vi "Main.vi"(11 "Module Admin":refnum<class "Delacor_lib_QMH_Module Admin.lvclass">) -> ()   [LabVIEW 2020, in "Acquisition.lvlib"]
doc: "This template is based off of the Queued Message Handler design pattern and the Queued Message Handler project template that ships with LabVIEW.\n\nThe main difference is that the queue is private to this module and communication between modules is performed via Broadcast and Request events.\n\nRequest events are wrapped in public API methods and are handled in the Event Handling Loop (EHL) of this VI. Any module can register for Broadcast events sent by this module. The EHL generates messages based on user interface actions.\n\nThe Message Handling Loop (MHL) processes messages generated by the EHL, or by other messages. The messages are string values, so new messages can be added easily to the Message Cases case structure in the MHL. Each message cluster can also provide an optional value for Message Data, which is a variant that can be converted to whatever message-specific data is required.\n_____\nBased on Delacor QMH Project Template 5.0.0.82."
uses:
  Acquisition.lvlib
  <vilib>/Delacor/Delacor QMH/Libraries/Module Admin_class/Delacor_lib_QMH_Module Admin.lvclass
  Module Data--cluster.ctl
  Stop Helper Loop Argument--cluster.ctl
  Stop Argument--cluster.ctl
  <vilib>/Delacor/Delacor QMH/Libraries/Message Queue_class/Delacor_lib_QMH_Message Queue.lvclass/Delacor_lib_QMH_Message Queue.ctl
  <vilib>/Delacor/Delacor QMH/Libraries/Module Admin_class/Delacor_lib_QMH_Module Admin.lvclass/Delacor_lib_QMH_Module Admin.ctl
  Start Acquire Argument--cluster.ctl
  Stop Acquire Argument--cluster.ctl
  <vilib>/Utility/miscctls.llb/LVPointTypeDef.ctl
  <vilib>/Delacor/Delacor QMH/Libraries/Message Queue_class/Delacor_lib_QMH_Enqueue Message (Single).vi
  <vilib>/Delacor/Delacor QMH/Libraries/Module Admin_class/Delacor_lib_QMH_Get External Launch.vi
  <vilib>/Utility/error.llb/Error Cluster From Error Code.vi
  <vilib>/ErrorRing/Error Ring.xnode
  <vilib>/Delacor/Delacor QMH/Libraries/Message Queue_class/Delacor_lib_QMH_Message Queue.lvclass
panel:
  out "Waveform Graph":dynamicdata(graph)
  out "error out":errorcluster
  out "Status":string
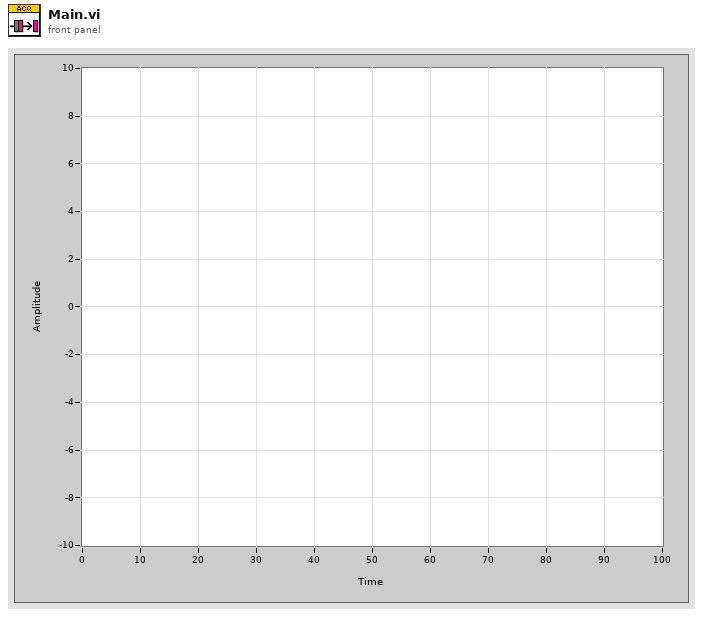
[diagram p1: front panel]
types:
  T1 = typedef "Acquisition.lvlib/Request Events--cluster.ctl" = cluster{"Stop Module":refnum<user-event>, "Show Panel":refnum<user-event>, "Hide Panel":refnum<user-event>, "Get Module Execution Status":refnum<user-event>, "Show Diagram":refnum<user-event>, "Start Helper Loop":refnum<user-event>, "Stop Helper Loop":refnum<user-event>, "Start Acquire":refnum<user-event>, "Stop Acquire":refnum<user-event>}
  T2 = typedef "Acquisition.lvlib/Module Data--cluster.ctl" = cluster{"Status":string}
  T3 = typedef "Acquisition.lvlib/Stop Helper Loop Argument--cluster.ctl" = cluster{"Boolean":bool}
  T4 = enum32{"invalid lock state", "Not Locked", "Locked (No Password)", "Password-protected"}
  T5 = typedef "Acquisition.lvlib/Stop Argument--cluster.ctl" = cluster{"Origin":string, "Exit via Stop Module Req?":bool, "Wait for Module to stop?":bool}
  T6 = typedef "Acquisition.lvlib/Start Acquire Argument--cluster.ctl" = cluster{"Boolean":bool}
  T7 = typedef "Acquisition.lvlib/Stop Acquire Argument--cluster.ctl" = cluster{"Boolean":bool}
  T8 = typedef "LVPointTypeDef.ctl" = cluster{"Horizontal":i16, "Vertical":i16}
  T9 = enum32{"Invalid", "Standard", "Closed", "Hidden", "Minimized", "Maximized"}
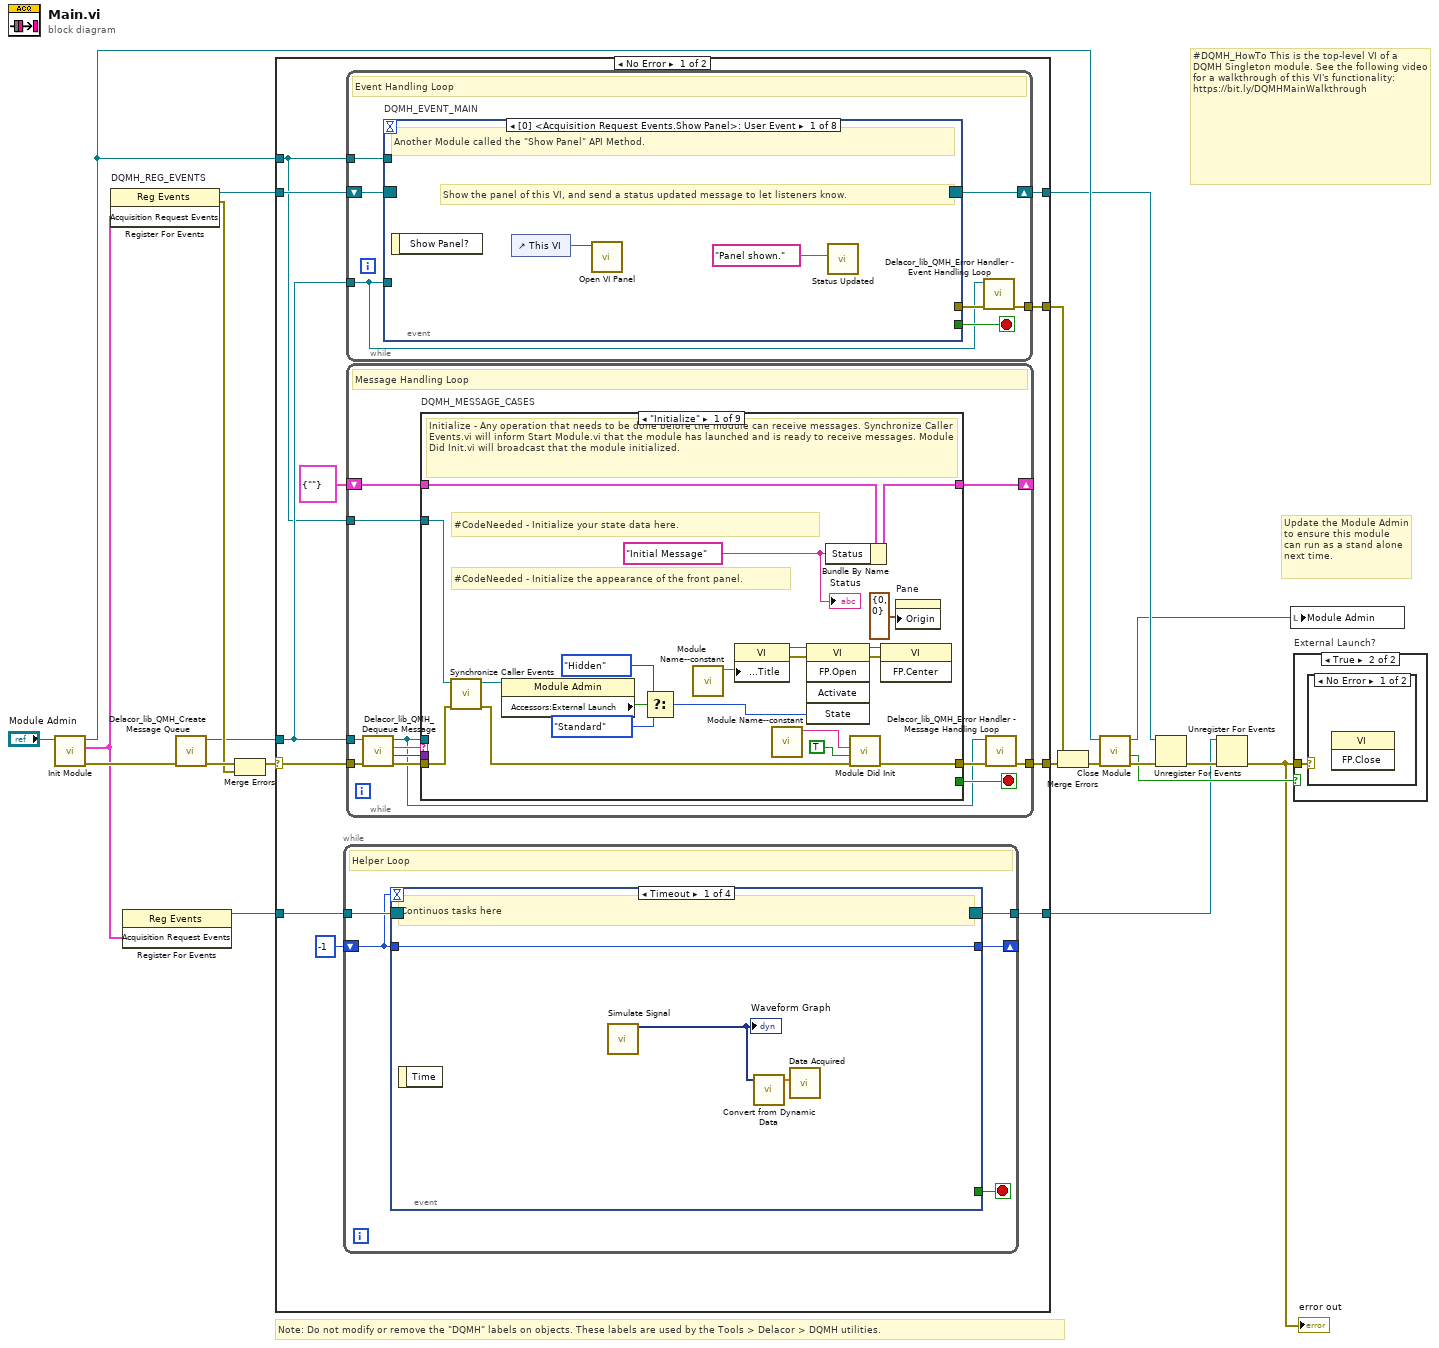
[diagram p0: block diagram]
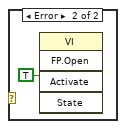
[diagram p3: hidden frame]
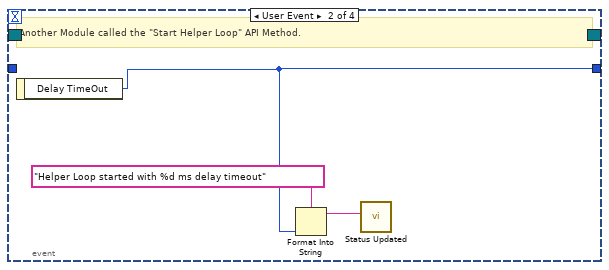
[diagram p4: hidden frame]
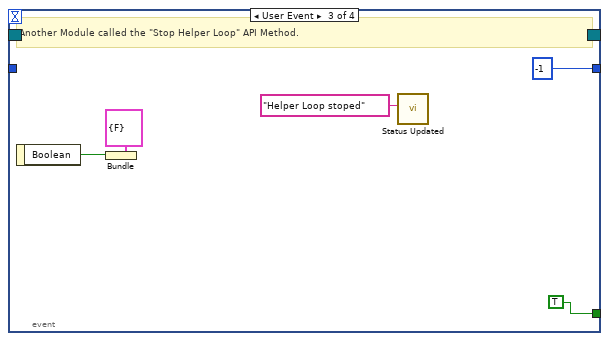
[diagram p5: hidden frame]
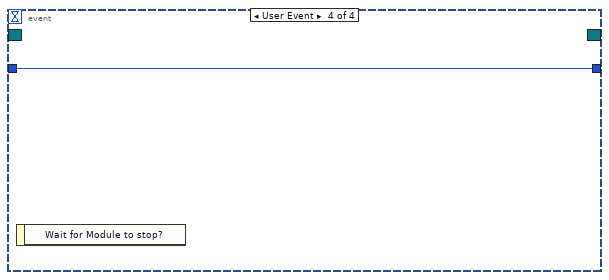
[diagram p6: hidden frame]
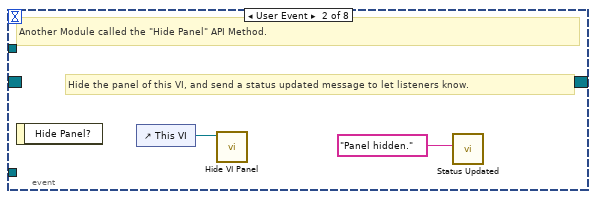
[diagram p7: hidden frame]
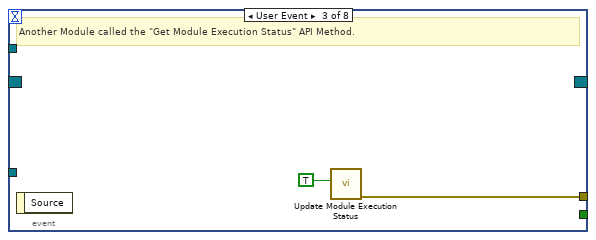
[diagram p8: hidden frame]
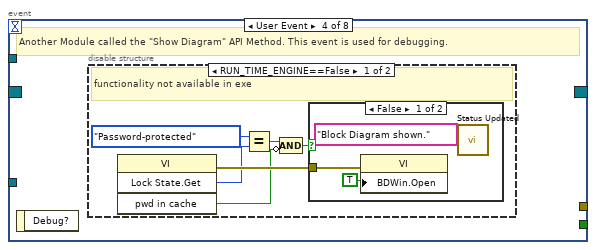
[diagram p9: hidden frame]
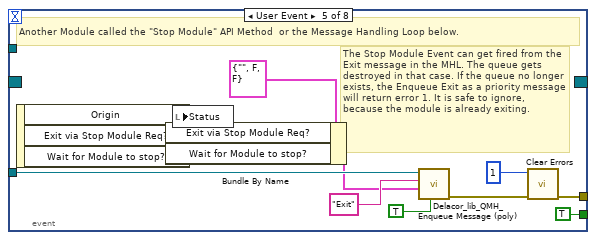
[diagram p12: hidden frame]
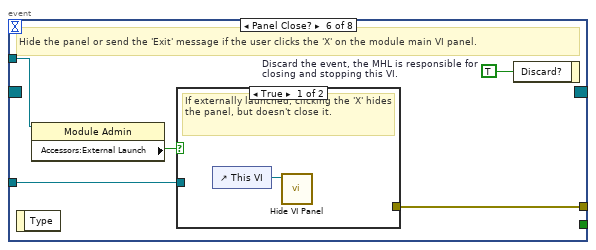
[diagram p13: hidden frame]
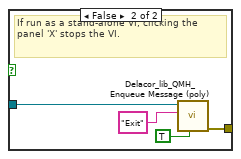
[diagram p14: hidden frame]
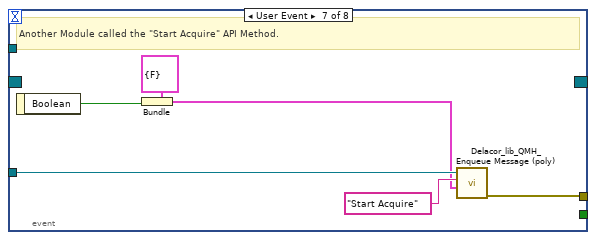
[diagram p15: hidden frame]
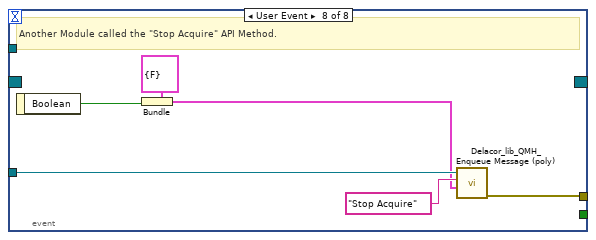
[diagram p16: hidden frame]
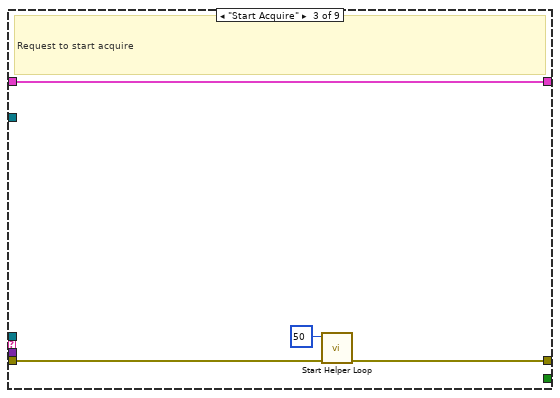
[diagram p18: hidden frame]
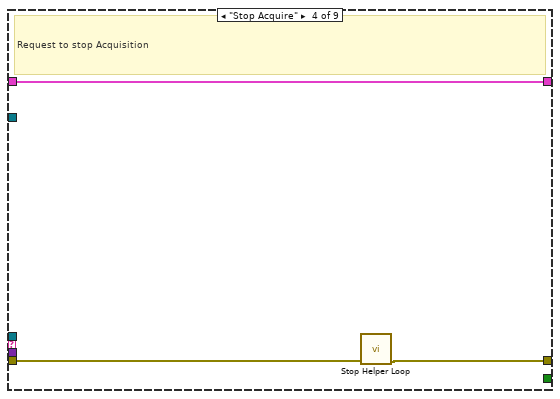
[diagram p19: hidden frame]
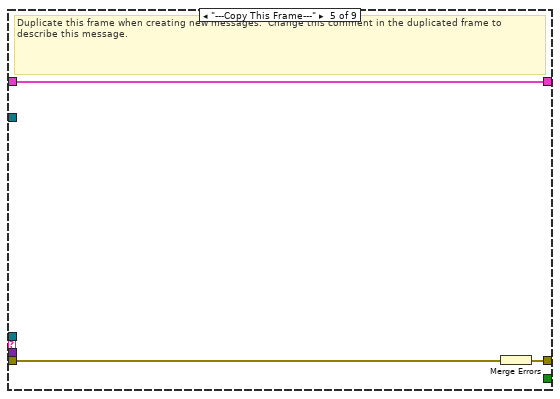
[diagram p20: hidden frame]
diagram:
  # "#DQMH_HowTo This is the top-level VI of a DQMH Singleton module. See the following video for a walkthrough of this VI's functionality: https://bit.ly/DQMHMainWalkthrough"
  # "Note: Do not modify or remove the \"DQMH\" labels on objects. These labels are used by the Tools > Delacor > DQMH utilities."
  # "Update the Module Admin to ensure this module can run as a stand alone next time."
  n1 = call "Init Module.vi"("Singleton Module Admin in"="Module Admin") -> ("error out"=w19:errorcluster, "Acquisition Request Events"=w3:T1, "Singleton Module Admin out"=w11:refnum<class "Delacor_lib_QMH_Module Admin.lvclass">)  [unwired: 8 in]
  n2 = register-events "DQMH_REG_EVENTS"(w3) -> (reference out=w9:refnum<event-registration>, error out=w12:errorcluster)  [unwired: 2 in]
  n3 = register-events(w3) -> (reference out=w4:refnum<event-registration>)  [unwired: 2 in, 1 out]
  n4 = call <vilib>:"Delacor_lib_QMH_Create Message Queue.vi"("error in (no error)"=w19) -> ("error out"=w14:errorcluster, "Message Queue"=w8:refnum<class "Delacor_lib_QMH_Message Queue.lvclass">)  [unwired: 9 in]
  n5 = Merge Errors(w14, w12) -> (w13:errorcluster)
  n6 = case shown="No Error" w13 {
    selector: w13 -> [w29 w199]
    tunnel: [w31 w198] -> w20
    tunnel: [w28 w204] -> w10
    tunnel: w9 -> [w26 w204]
    tunnel: w8 -> [w25 w197]
    tunnel: [w30 _] -> w17
    tunnel: w11 -> [w24 w200]
    tunnel: w4 -> [w23 _]
    tunnel: [w22 _] -> w1
    frame No Error {
      n7 = while {
        tunnel: w23 -> [w36]
        tunnel: [w35] -> w22
        shift-right: [w34] -> _
        shift-left: -1 -> [w33]
        stop <- w32 stop-if-true
        # "Helper Loop"
        n8 = event shown="[0] Timeout" {
          selector: w36 -> [_ _ _ _]
          dyn-events: [_ _ _ _] -> w35
          timeout: w33 -> [_ _ _ _]
          tunnel: [w39 w41 -1 w48] -> w34
          tunnel: w33 -> [w39 _ _ w48]
          tunnel: [_ _ TRUE _] -> w32
          event Timeout {
            # "Continuos tasks here"
            n9 = event-data() -> ()  [unwired: 1 in, 1 out]
            n10 = call "Simulate Signal"() -> ("Sine"=w38:dynamicdata)  [unwired: 14 in, 1 out]
            "Waveform Graph" <- w38
            n11 = call "Convert from Dynamic Data"("Dynamic Data Type"=w38) -> ("Array"=w37:dbl[])  [unwired: 3 in]
            n12 = call "Data Acquired.vi"("Data"=w37) -> ()  [unwired: 10 in, 1 out]
          }
          event User Event {
            # "Another Module called the \"Start Helper Loop\" API Method."
            n13 = event-data() -> ("Delay TimeOut"=w41:i32)  [unwired: 1 in]
            n14 = Format Into String(format string="Helper Loop started with %d ms delay timeout", w41) -> (resulting string=w42:string)  [unwired: 2 in, 1 out]
            n15 = call "Status Updated.vi"("Status"=w42) -> ()  [unwired: 10 in, 1 out]
          }
          event User Event {
            # "Another Module called the \"Stop Helper Loop\" API Method."
            n16 = event-data() -> ("Boolean"=w46:bool)  [unwired: 1 in]
            n17 = Bundle(cluster=T3 {"Boolean"=FALSE} ("Stop Helper Loop Argument"), "Boolean"=w46) -> ()  [unwired: 1 out]
            n18 = call "Status Updated.vi"("Status"="Helper Loop stoped") -> ()  [unwired: 10 in, 1 out]
          }
          event User Event {
            n19 = event-data() -> ()  [unwired: 1 in, 1 out]
          }
        }
      }
      n20 = while {
        tunnel: w25 -> [w49]
        shift-right: [w52] -> w28
        shift-left: w26 -> [w53]
        tunnel: [w54] -> w30
        tunnel: w24 -> [w50]
        stop <- w51 stop-if-true
        # "Event Handling Loop"
        n21 = event "DQMH_EVENT_MAIN" shown="[0] <Acquisition Request Events.Show Panel>: User Event" {
          selector: w53 -> [_ _ _ _ _ _ _ _]
          dyn-events: [_ _ _ _ _ _ _ _] -> w52
          timeout: _ -> [_ _ _ _ _ _ _ _]
          tunnel: [_ _ _ _ TRUE ("Discard?") _ _ _] -> w51
          tunnel: w49 -> [_ _ _ _ w78 w85 w98 w104]
          tunnel: [_ _ w61 _ w81 w87 w93 w99] -> w55
          tunnel: w50 -> [_ _ _ _ _ w84 _ _]
          event User Event {
            # "Show the panel of this VI, and send a status updated message to let listeners know."
            # "Another Module called the \"Show Panel\" API Method."
            n22 = event-data() -> ()  [unwired: 1 in, 1 out]
            n23 = control-ref of="This VI"() -> (w57:refnum<vi>)
            n24 = call "Open VI Panel.vi"("VI"=w57) -> ()  [unwired: 10 in, 1 out]
            n25 = call "Status Updated.vi"("Status"="Panel shown." ("format string")) -> ()  [unwired: 10 in, 1 out]
          }
          event User Event {
            # "Hide the panel of this VI, and send a status updated message to let listeners know."
            # "Another Module called the \"Hide Panel\" API Method."
            n26 = event-data() -> ()  [unwired: 1 in, 1 out]
            n27 = control-ref of="This VI"() -> (w59:refnum<vi>)
            n28 = call "Hide VI Panel.vi"("VI"=w59) -> ()  [unwired: 10 in, 1 out]
            n29 = call "Status Updated.vi"("Status"="Panel hidden." ("format string")) -> ()  [unwired: 10 in, 1 out]
          }
          event User Event {
            # "Another Module called the \"Get Module Execution Status\" API Method."
            n30 = event-data() -> ()  [unwired: 1 in, 1 out]
            n31 = call "Update Module Execution Status.vi"("Running?"=TRUE) -> ("error out"=w61:errorcluster)  [unwired: 10 in]
          }
          event User Event {
            # "Another Module called the \"Show Diagram\" API Method. This event is used for debugging."
            n32 = event-data() -> ()  [unwired: 1 in, 1 out]
            n33 = disable-structure shown="RUN_TIME_ENGINE==False" {
              frame condition #0 (active) {
                # "functionality not available in exe"
                n34 = invoke class="VI" method="Lock State.Get"() -> (error out=w67:errorcluster, "Get Lock State"=w66:T4, "pwd in cache"=w63:bool)  [unwired: 4 in, 1 out]
                n35 = Equal?(x=T4."Password-protected", y=w66) -> (x = y?=w64:bool)
                n36 = Compound Arithmetic op=AND(w64, invert w63) -> (w62:bool)
                n37 = case shown="False" w62 {
                  tunnel: w67 -> [w70 _]
                  frame False {
                    n38 = property class="VI"(error in=w70, "BDWin.Open"=TRUE ("Block Diagram Window:Open")) -> ()  [unwired: 1 in, 2 out]
                    n39 = call "Status Updated.vi"("Status"="Block Diagram shown." ("format string")) -> ()  [unwired: 10 in, 1 out]
                  }
                  frame True {
                    # "Password-protected VI, and the password is not in the cache. Do not show the diagram."
                  }
                }
              }
              frame condition #1 {
              }
            }
          }
          event User Event {
            # "The Stop Module Event can get fired from the Exit message in the MHL. The queue gets destroyed in that case. If the queue no longer exists, the Enqueue Exit as a priority message will return error 1. It is safe to ignore, because the module is already exiting."
            # "Another Module called the \"Stop Module\" API Method  or the Message Handling Loop below."
            n40 = event-data() -> ("Origin"=w77:string, "Exit via Stop Module Req?"=w73:bool, "Wait for Module to stop?"=w72:bool)  [unwired: 1 in]
            n41 = Bundle By Name(cluster=T5 {"Origin"="", "Exit via Stop Module Req?"=FALSE, "Wait for Module to stop?"=FALSE} ("Stop Argument"), "Exit via Stop Module Req?"=w73, "Wait for Module to stop?"=w72) -> (w71:T5)
            n42 = local write "Status"(w77) -> ()
            n43 = call-poly <vilib>:"Delacor_lib_QMH_Enqueue Message (poly).vi"("Priority Message? (F)"=TRUE, "Message Data"=w71, "Message"="Exit", "Message Queue in"=w78) -> ("error out"=w82:errorcluster)  [unwired: 6 in, 1 out]
            n44 = call <vilib>:"Clear Errors.vi"("error in (no error)"=w82, "specific error code to clear (0: all)"=1) -> ("error out"=w81:errorcluster)  [unwired: 4 in, 1 out]
          }
          event Panel Close? {
            w86 = TRUE  # Discard the event, the MHL is responsible for closing and stopping this VI.
            # "Hide the panel or send the 'Exit' message if the user clicks the 'X' on the module main VI panel."
            n45 = event-data() -> ()  [unwired: 1 in, 1 out]
            n46 = property class="Module Admin"(reference=w84) -> ("Accessors:External Launch"=w83:bool)  [unwired: 1 in, 2 out]
            n47 = case shown="True" w83 {
              tunnel: w85 -> [_ w91]
              tunnel: [_ w92] -> w87
              frame True {
                # "If externally launched, clicking the 'X' hides the panel, but doesn't close it."
                n48 = control-ref of="This VI"() -> (w88:refnum<vi>)
                n49 = call "Hide VI Panel.vi"("VI"=w88) -> ()  [unwired: 10 in, 1 out]
              }
              frame False {
                # "If run as a stand-alone VI, clicking the panel 'X' stops the VI."
                n50 = call-poly <vilib>:"Delacor_lib_QMH_Enqueue Message (poly).vi"("Priority Message? (F)"=TRUE, "Message"="Exit", "Message Queue in"=w91) -> ("error out"=w92:errorcluster)  [unwired: 7 in, 1 out]
              }
            }
            n51 = event-data("Discard?"=w86) -> ()  [unwired: 1 in, 1 out]
          }
          event User Event {
            # "Another Module called the \"Start Acquire\" API Method."
            n52 = event-data() -> ("Boolean"=w94:bool)  [unwired: 1 in]
            n53 = Bundle(cluster=T6 {"Boolean"=FALSE} ("Start Acquire Argument"), "Boolean"=w94) -> (w95:T6)
            n54 = call-poly <vilib>:"Delacor_lib_QMH_Enqueue Message (poly).vi"("Message Data"=w95, "Message"="Start Acquire", "Message Queue in"=w98) -> ("error out"=w93:errorcluster)  [unwired: 7 in, 1 out]
          }
          event User Event {
            # "Another Module called the \"Stop Acquire\" API Method."
            n55 = event-data() -> ("Boolean"=w100:bool)  [unwired: 1 in]
            n56 = Bundle(cluster=T7 {"Boolean"=FALSE} ("Stop Acquire Argument"), "Boolean"=w100) -> (w101:T7)
            n57 = call-poly <vilib>:"Delacor_lib_QMH_Enqueue Message (poly).vi"("Message Data"=w101, "Message"="Stop Acquire", "Message Queue in"=w104) -> ("error out"=w99:errorcluster)  [unwired: 7 in, 1 out]
          }
        }
        n58 = call-dynamic "Delacor_lib_QMH_Error Handler - Event Handling Loop.vi"("error in (no error)"=w55, "Message Queue in"=w49) -> ("dup error in"=w54:errorcluster)  [unwired: 8 in, 1 out]
      }
      n59 = while {
        tunnel: w25 -> [w107]
        shift-right: [w111] -> _
        shift-left: T2 {"Status"=""} ("Data Cluster") -> [w112]
        tunnel: w29 -> [w115]
        tunnel: [w113] -> w31
        tunnel: w24 -> [w105]
        stop <- w110 stop-if-true
        # "Message Handling Loop"
        n60 = call-dynamic "Delacor_lib_QMH_Dequeue Message.vi"("error in (no error)"=w115, "Message Queue in"=w107) -> ("error out"=w114:errorcluster, "Message Data"=w108:variant, "Message"=w109:string, "Message Queue out"=w106:refnum<class "Delacor_lib_QMH_Message Queue.lvclass">)  [unwired: 6 in]
        n61 = case "DQMH_MESSAGE_CASES" shown="\"Initialize\"" w109 {
          selector: w109 -> [_ _ _ _ _ _ _ _ w184]
          tunnel: w106 -> [_ _ _ _ _ _ w154 w176 _]
          tunnel: w114 -> [w134 w138 w141 w144 w148 w150 w161 w182 w186]
          tunnel: [w132 w138 w140 w143 w147 w150 w157 w179 w187] -> w116
          tunnel: w112 -> [w123 w137 w142 w145 w146 w149 w156 w175 w185]
          tunnel: [w122 w137 w142 w145 w146 w149 w156 w175 w185] -> w111
          tunnel: [_ _ _ _ _ _ _ w174 _] -> w110
          tunnel: w108 -> [_ _ _ _ _ _ w155 w173 _]
          tunnel: w105 -> [w124 _ _ _ _ _ w153 w168 _]
          frame "Initialize" {
            w117 = "Initial Message" ("Initial Message")
            # "#CodeNeeded - Initialize the appearance of the front panel."
            # "#CodeNeeded - Initialize your state data here."
            # "Initialize - Any operation that needs to be done before the module can receive messages. Synchronize Caller Events.vi will inform Start Module.vi that the module has launched and is ready to receive messages. Module Did Init.vi will broadcast that the module initialized."
            n62 = call "Synchronize Caller Events.vi"("error in (no error)"=w134, "Singleton Module Admin in"=w124) -> ("error out"=w133:errorcluster, "Singleton Module Admin out"=w119:refnum<class "Delacor_lib_QMH_Module Admin.lvclass">)  [unwired: 8 in]
            n63 = property class="Module Admin"(reference=w119) -> ("Accessors:External Launch"=w128:bool)  [unwired: 1 in, 2 out]
            n64 = Select(t=T9."Hidden" ("State"), s=w128, f=T9."Standard" ("State")) -> (s? t:f=w125:T9)
            n65 = call "Module Name--constant.vi"() -> ("Module Name"=w131:string)  [unwired: 11 in]
            n66 = property class="VI"("Front Panel.Title"=w131) -> (reference out=w130:refnum<vi>, error out=w136:errorcluster)  [unwired: 2 in]
            n67 = call "Module Name--constant.vi"() -> ("Module Name"=w120:string)  [unwired: 11 in]
            n68 = invoke class="VI" method="FP.Open"(reference=w130, error in=w136, "State"=w125) -> (reference out=w129:refnum<vi>, error out=w135:errorcluster)  [unwired: 2 in, 3 out]
            n69 = Bundle By Name(cluster=w123, "Status"=w117) -> (w122:T2)
            n70 = call "Module Did Init.vi"("error in (no error)"=w133, "Initialized?"=TRUE, "Origin"=w120) -> ("error out"=w132:errorcluster)  [unwired: 8 in]
            n71 = invoke class="VI" method="FP.Center"(reference=w129, error in=w135) -> ()  [unwired: 1 in, 3 out]
            n72 = property on="Pane" class="Pane"("Origin"=T8 {"Horizontal"=0, "Vertical"=0}) -> ()  [unwired: 2 in, 2 out]
            "Status" <- w117
          }
          frame "--- Module Specific ---" {
            # "Separator -- The following cases handle messages specific to this Module."
          }
          frame "Start Acquire" {
            # "Request to start acquire"
            n73 = call "Start Helper Loop.vi"("error in (no error)"=w141, "Delay TimeOut"=50) -> ("error out"=w140:errorcluster)  [unwired: 9 in]
          }
          frame "Stop Acquire" {
            # "Request to stop Acquisition"
            n74 = call "Stop Helper Loop.vi"("error in (no error)"=w144) -> ("error out"=w143:errorcluster)  [unwired: 10 in]
          }
          frame "---Copy This Frame---" {
            # "Duplicate this frame when creating new messages.  Change this comment in the duplicated frame to describe this message."
            n75 = Merge Errors(w148) -> (w147:errorcluster)
          }
          frame "--- Exit and Error Handling---" {
            # "Separator - The following cases handle errors and exit messages."
          }
          frame "Error" {
            # "#CodeRecommended - If you ever change the name of this \"Error\" message, you'll need to update the name in the Check Loop Error.vi as well."
            # "#CodeRecommended - If the module is running in standalone mode (External Launch = FALSE), this code will pop up an error dialog and call the 'Exit' message if an error occurs. Add more fine-grained error handling here."
            # "Error - Check the error message data and respond accordingly. This message is sent by the \"Error Handler\" VIs at the end of each loop in this application."
            n76 = property class="Module Admin"(reference=w153) -> ("Accessors:External Launch"=w152:bool)  [unwired: 1 in, 2 out]
            n77 = Variant To Data(error in=w161, type=errorcluster {"status"=FALSE, "code"=0, "source"=""} ("error constant"), Variant=w155) -> (data=w162:errorcluster, error out=w159:errorcluster)
            n78 = call "Module Name--constant.vi"() -> ("Module Name"=w151:string)  [unwired: 11 in]
            n79 = call "Error Reported.vi"("Additional Information"=w151, "Error"=w162) -> ()  [unwired: 9 in, 1 out]
            n80 = case shown="False" w152 {
              tunnel: [w167 _] -> w158
              tunnel: w154 -> [w165 _]
              tunnel: w162 -> [w166 _]
              frame False {
                # "If the module is running standalone, then pop up an error dialog and call the \"Exit\" message."
                n81 = call <vilib>:"Simple Error Handler.vi"("error in (no error)"=w166) -> ()  [unwired: 4 in, 5 out]
                n82 = call-poly <vilib>:"Delacor_lib_QMH_Enqueue Message (poly).vi"("Priority Message? (F)"=TRUE, "Message"="Exit", "Message Queue in"=w165) -> ("error out"=w167:errorcluster)  [unwired: 7 in, 1 out]
              }
              frame True {
                # "If the module was launched externally, calling the Error Reported broadcast VI is the only action performed by the \"Error\" message. The module's caller can then process the error appropriately."
              }
            }
            n83 = Merge Errors(w159, w158) -> (w157:errorcluster)
            n84 = local write "error out"(w157) -> ()
          }
          frame "Exit" {
            w172 = 91  # 91: not all Exit messages will have an argument
            w174 = TRUE  # Stop the VI
            # "Release the message queue reference"
            # "#CodeNeeded - Add any required cleanup code here"
            # "Exit - Exit the application."
            n85 = Variant To Data(error in=w182, type=T5 {"Origin"="", "Exit via Stop Module Req?"=FALSE, "Wait for Module to stop?"=FALSE} ("Stop Argument"), Variant=w173) -> (data=w170:T5, error out=w178:errorcluster)
            n86 = call <vilib>:"Clear Errors.vi"("error in (no error)"=w178, "specific error code to clear (0: all)"=w172) -> ("error out"=w181:errorcluster)  [unwired: 4 in, 1 out]
            n87 = control-ref of="This VI"() -> (w169:refnum<vi>)
            n88 = call-dynamic "Delacor_lib_QMH_Release Message Queue.vi"("error in (no error)"=w181, "Message Queue"=w176) -> ("error out"=w180:errorcluster)  [unwired: 9 in]
            n89 = call "Handle Exit.vi"("Stop Argument"=w170, "Admin in"=w168, "VI reference"=w169) -> ("error out"=w177:errorcluster)  [unwired: 7 in, 1 out]
            n90 = Merge Errors(w180, w177) -> (w179:errorcluster)
          }
          frame Default {
            # "'Default' case only runs if there is a message that isn't defined in any of the other cases.  Output a programming error."
            n91 = call "Module Name--constant.vi"() -> ("Module Name"=w183:string)  [unwired: 11 in]
            n92 = xnode "Error Ring"("parameter 0"=w184, "parameter 1"=w183) -> ("error out"=w188:errorcluster)
            n93 = Merge Errors(w186, w188) -> (w187:errorcluster)
          }
        }
        n94 = call-dynamic "Delacor_lib_QMH_Error Handler - Message Handling Loop.vi"("error in (no error)"=w116, "Message Queue in"=w106) -> ("dup error in"=w113:errorcluster)  [unwired: 8 in, 1 out]
      }
    }
    frame Error {
      # "Synchronize Caller Events.vi will inform Start Module.vi that the module has launched and will let the code calling Start Module.vi register for broadcasts and would permit the caller receive the broadcast that an error occurred at launch time."
      n95 = call-dynamic "Delacor_lib_QMH_Release Message Queue.vi"("error in (no error)"=w199, "Message Queue"=w197) -> ("error out"=w198:errorcluster)  [unwired: 9 in]
      n96 = call "Synchronize Caller Events.vi"("Singleton Module Admin in"=w200) -> ("error out"=w205:errorcluster)  [unwired: 9 in, 1 out]
      n97 = call "Module Name--constant.vi"() -> ("Module Name"=w203:string)  [unwired: 11 in]
      n98 = Format Into String(format string="An error occurred during initialization. %s is no longer running.", w203) -> (resulting string=w201:string)  [unwired: 2 in, 1 out]
      n99 = Merge Errors(w198, w205) -> (w206:errorcluster)
      n100 = call "Error Reported.vi"("Additional Information"=w201, "Error"=w206) -> ()  [unwired: 9 in, 1 out]
    }
  }
  n101 = Merge Errors(w17, w20) -> (w16:errorcluster)
  n102 = call "Close Module.vi"("error in (no error)"=w16, "Module Admin in"=w11) -> ("error out"=w18:errorcluster, "External Launch"=w5:bool, "Module Admin out"=w6:refnum<class "Delacor_lib_QMH_Module Admin.lvclass">)  [unwired: 7 in]
  n103 = Unregister For Events(event registration refnum=w10, error in=w18) -> (error out=w15:errorcluster)
  n104 = Unregister For Events(event registration refnum=w1, error in=w15) -> (error out=w2:errorcluster)
  "error out" <- w2
  n105 = local write "Module Admin"(w6) -> ()
  n106 = case "External Launch?" shown="True" w5 {
    tunnel: w2 -> [_ w207]
    frame False {
    }
    frame True {
      n107 = case shown="No Error" w207 {
        frame No Error {
          n108 = invoke class="VI" method="FP.Close"() -> ()  [unwired: 3 in, 3 out]
        }
        frame Error {
          n109 = invoke class="VI" method="FP.Open"("Activate"=TRUE ("Activate?")) -> ()  [unwired: 4 in, 5 out]
        }
      }
    }
  }
